vi "srednia biegnaca.vi"() -> ()   [LabVIEW 2014]
panel:
  out "Œrednia":dbl
  out "Ostatnia wartoœæ":dbl
  out "Waveform Chart 2":cluster{"number: 0 to 1":dbl, dbl}(graph)
  in  "stop 2":bool
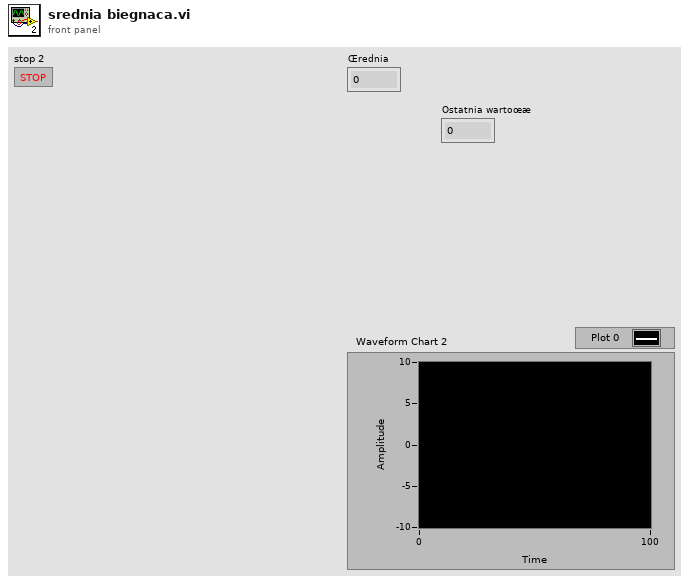
[diagram p1: front panel]
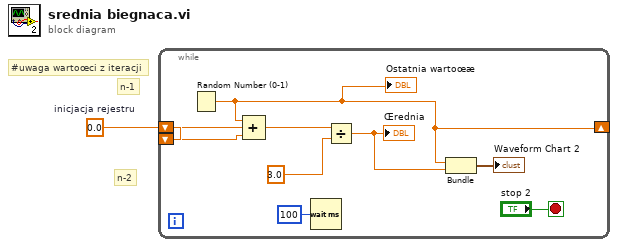
[diagram p0: block diagram]
diagram:
  w1 = 0.0  # inicjacja rejestru
  # "n-2"
  # "n-1"
  # "#uwaga wartoœci z iteracji"
  n1 = while {
    shift-right: [w6] -> _
    shift-left: w1 -> [w10]
    shift-left: w1 -> [w9]
    stop <- "stop 2" stop-if-true
    n2 = Random Number (0-1)() -> (number: 0 to 1=w6:dbl)
    "Ostatnia wartoœæ" <- w6
    n3 = Compound Arithmetic op=ADD(w6, w10, w9) -> (w8:dbl)
    n4 = Wait (ms)(milliseconds to wait=u32 100) -> ()  [unwired: 1 out]
    n5 = Divide(x=w8, y=3.0) -> (x/y=w5:dbl)
    "Œrednia" <- w5
    n6 = Bundle "Bundle"("number: 0 to 1"=w6, w5) -> (→"Waveform Chart 2":cluster{"number: 0 to 1":dbl, dbl})  [unwired: 1 in]
  }
